vi "TeleopLogic.vi"() -> ()   [LabVIEW 2018]
uses:
  <vilib>/Rock Robotics/WPI/Utilities/WPI_GetSetVariantRefNum.vi
  Globals.vi
panel:
  out "CancelZeroHatch":bool
  # "Copilot controls:\nRight button: set arm out\nRight switch: hold down to release hatch from hatch catch\nLeft button: set arm in\nLeft switch: Cargo out?\nA button: lift low\nB button: lift mid\nY button: lift high\nRight joystick button: Start automated climb sequence\nRight joystick y axis: Up/down all climb actuators\nLeft joystick y axis: Move forward climbing\nPOV hat right: Up front climb actuator\nPOV hat left: Up back climb actuators"
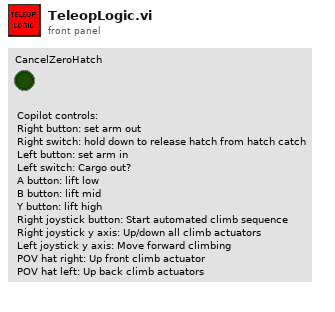
[diagram p1: front panel]
types:
  T1 = typedef "WPI_JoystickDevRef.ctl" = cluster{"Device":T2}
  T2 = typedef "WPI_JoystickDeviceEnum.ctl" = enum16{"USB 0", "USB 1", "USB 2", "USB 3", "USB 4", "USB 5"}
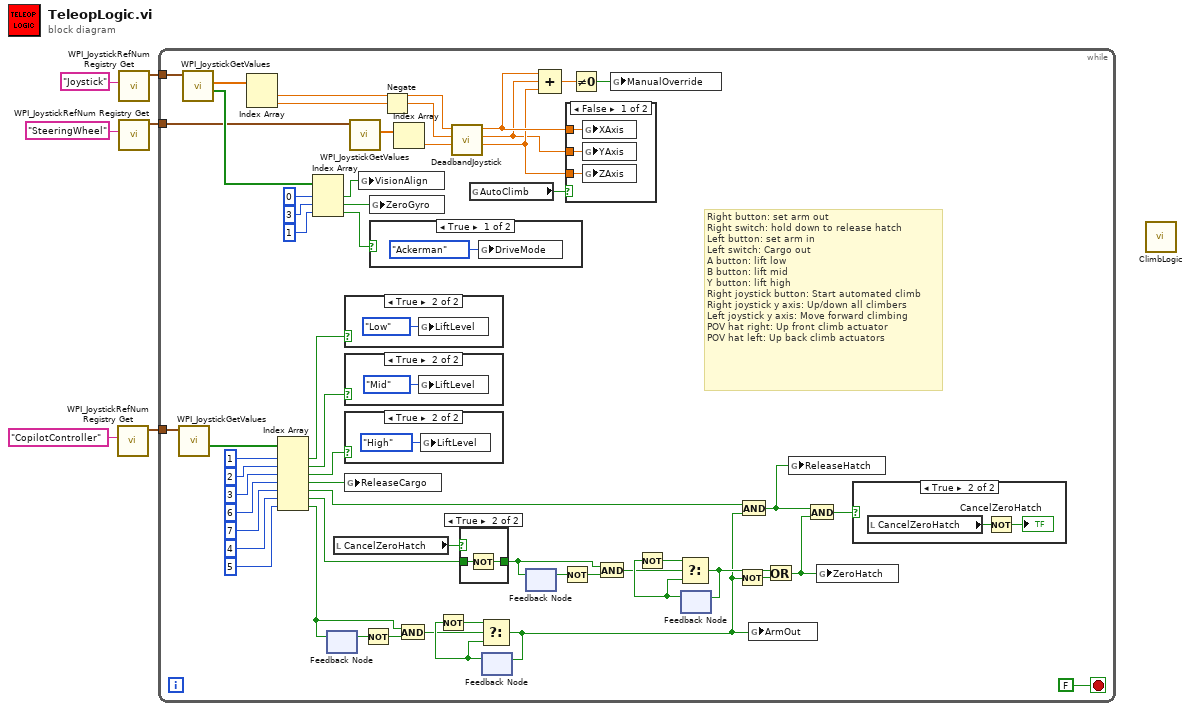
[diagram p0: block diagram]
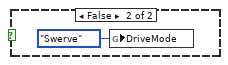
[diagram p8: hidden frame]
diagram:
  n1 = call <vilib>:"WPI_JoystickRefNum Registry Get.vi"("refnum name"="CopilotController") -> ("JoystickDevRef"=w1:T1)  [unwired: 1 in, 9 out]
  n2 = call <vilib>:"WPI_JoystickRefNum Registry Get.vi"("refnum name"="Joystick") -> ("JoystickDevRef"=w3:T1)  [unwired: 1 in, 9 out]
  n3 = call <vilib>:"WPI_JoystickRefNum Registry Get.vi"("refnum name"="SteeringWheel") -> ("JoystickDevRef"=w2:T1)  [unwired: 1 in, 9 out]
  n4 = while {
    tunnel: w3 -> [w51]
    tunnel: w2 -> [w50]
    tunnel: w1 -> [w49]
    stop <- FALSE stop-if-true
    # "Right button: set arm out\nRight switch: hold down to release hatch\nLeft button: set arm in\nLeft switch: Cargo out\nA button: lift low\nB button: lift mid\nY button: lift high\nRight joystick button: Start automated climb\nRight joystick y axis: Up/down all climbers\nLeft joystick y axis: Move forward climbing\nPOV hat right: Up front climb actuator\nPOV hat left: Up back climb actuators"
    n5 = call <vilib>:"WPI_JoystickGetValues.vi"("JoystickDevRef"=w49) -> ("Buttons"=w32:bool[])  [unwired: 6 in, 4 out]
    n6 = call <vilib>:"WPI_JoystickGetValues.vi"("JoystickDevRef"=w51) -> ("Buttons"=w59:bool[], "Axes"=w61:dbl[])  [unwired: 6 in, 3 out]
    n7 = Index Array(array=w61) -> (element #1=w9:dbl, element #2=w60:dbl)  [unwired: 2 in]
    n8 = Index Array(array=w32, index #1=1 ("index"), index #2=2 ("index"), index #3=3 ("index"), index #4=6 ("index"), index #5=7 ("index"), index #6=4 ("index"), index #7=5 ("index")) -> (element #1=w38:bool, element #2=w37:bool, element #3=w36:bool, element #4=w35:bool, element #5=w24:bool, element #6=w22:bool, element #7=w26:bool)
    n9 = Index Array(array=w59, index #1=0 ("index"), index #2=3 ("index"), index #3=1 ("index")) -> (element #1=w55:bool, element #2=w52:bool, element #3=w56:bool)
    n10 = feedback #1() -> (w27:bool)  [unwired: 1 in]
    n11 = feedback-in #1(w26) -> ()
    n12 = local read "CancelZeroHatch"() -> (w23:bool)
    n13 = case shown="True" w38 {
      frame False {
      }
      frame True {
        n14 = global write "Globals.vi" "LiftLevel"(enum16{"Low", "Mid", "High"}."Low" ("LiftLevel")) -> ()
      }
    }
    n15 = case shown="True" w37 {
      frame False {
      }
      frame True {
        n16 = global write "Globals.vi" "LiftLevel"(enum16{"Low", "Mid", "High"}."Mid" ("LiftLevel")) -> ()
      }
    }
    n17 = case shown="True" w36 {
      frame False {
      }
      frame True {
        n18 = global write "Globals.vi" "LiftLevel"(enum16{"Low", "Mid", "High"}."High" ("LiftLevel")) -> ()
      }
    }
    n19 = global write "Globals.vi" "ReleaseCargo"(w35) -> ()
    n20 = call <vilib>:"WPI_JoystickGetValues.vi"("JoystickDevRef"=w50) -> ("Axes"=w62:dbl[])  [unwired: 6 in, 4 out]
    n21 = global write "Globals.vi" "VisionAlign"(w55) -> ()
    n22 = Not(x=w27) -> (.not. x?=w28:bool)
    n23 = global write "Globals.vi" "ZeroGyro"(w52) -> ()
    n24 = case shown="True" w56 {
      frame True {
        n25 = global write "Globals.vi" "DriveMode"(enum16{"Swerve", "Ackerman"}."Ackerman" ("DriveMode")) -> ()
      }
      frame False {
        n26 = global write "Globals.vi" "DriveMode"(enum16{"Swerve", "Ackerman"}."Swerve" ("DriveMode")) -> ()
      }
    }
    n27 = Negate(x=w60) -> (-x=w8:dbl)
    n28 = Index Array(array=w62) -> (element=w53:dbl)  [unwired: 1 in]
    n29 = And(x=w26, y=w28) -> (x .and. y?=w29:bool)
    n30 = call "DeadbandJoystick.vi"("Z"=w53, "Y"=w8, "X"=w9) -> ("Z'"=w42:dbl, "Y'"=w41:dbl, "X'"=w43:dbl)  [unwired: 6 in]
    n31 = case shown="True" w23 {
      tunnel: [w66 w67] -> w16
      tunnel: w22 -> [w66 w68]
      frame False {
      }
      frame True {
        n32 = Not(x=w68) -> (.not. x?=w67:bool)
      }
    }
    n33 = global read "Globals.vi" "AutoClimb"() -> (w7:bool)
    n34 = feedback #2() -> (w30:bool)  [unwired: 1 in]
    n35 = Not(x=w30) -> (.not. x?=w31:bool)
    n36 = Select(t=w31, s=w29, f=w30) -> (s? t:f=w13:bool)
    n37 = feedback-in #2(w13) -> ()
    n38 = feedback #3() -> (w17:bool)  [unwired: 1 in]
    n39 = feedback-in #3(w16) -> ()
    n40 = Compound Arithmetic op=ADD(w43, w41, w42) -> (w40:dbl)
    n41 = Not(x=w17) -> (.not. x?=w18:bool)
    n42 = case shown="False" w7 {
      tunnel: w43 -> [w65 _]
      tunnel: w42 -> [w64 _]
      tunnel: w41 -> [w63 _]
      frame False {
        n43 = global write "Globals.vi" "XAxis"(w65) -> ()
        n44 = global write "Globals.vi" "YAxis"(w63) -> ()
        n45 = global write "Globals.vi" "ZAxis"(w64) -> ()
      }
      frame True {
      }
    }
    n46 = Not Equal To 0?(x=w40) -> (x != 0?=w39:bool)
    n47 = And(x=w16, y=w18) -> (x .and. y?=w19:bool)
    n48 = global write "Globals.vi" "ManualOverride"(w39) -> ()
    n49 = feedback #4() -> (w20:bool)  [unwired: 1 in]
    n50 = Not(x=w20) -> (.not. x?=w21:bool)
    n51 = Select(t=w21, s=w19, f=w20) -> (s? t:f=w15:bool)
    n52 = feedback-in #4(w15) -> ()
    n53 = Not(x=w13) -> (.not. x?=w25:bool)
    n54 = And(x=w24, y=w13) -> (x .and. y?=w11:bool)
    n55 = global write "Globals.vi" "ArmOut"(w13) -> ()
    n56 = Or(x=w15, y=w25) -> (x .or. y?=w10:bool)
    n57 = global write "Globals.vi" "ReleaseHatch"(w11) -> ()
    n58 = And(x=w11, y=w10) -> (x .and. y?=w12:bool)
    n59 = global write "Globals.vi" "ZeroHatch"(w10) -> ()
    n60 = case shown="True" w12 {
      frame False {
      }
      frame True {
        n61 = local read "CancelZeroHatch"() -> (w70:bool)
        n62 = Not(x=w70) -> (.not. x?=→"CancelZeroHatch":bool)
      }
    }
  }
  n63 = call "ClimbLogic.vi"() -> ()  [unwired: 12 in]
